vi "Demo.vi"() -> (4 "图像时间戳":u32=16532020 format="%_32g")   [LabVIEW 2012]
uses:
  MVCAMSDK.dll
panel:
  in  "自定义分辨率设置":bool
  in  "ROI分辨率":T1
  in  "预设分辨率设置":bool
  in  "预设分辨率":T2(radio)
  out "帧速":u32
  out "帧间耗时\n单位：（0.1ms）":u32
  in  "相机枚举":T3(ring)
  in  "自动曝光模式":bool=TRUE caption="软触发"
  in  "手动曝光模式":bool caption="软触发"
  in  "曝光时间，单位微秒":dbl=11000.0 format="%#_6f"
  in  "硬触发模式":bool caption="软触发"
  in  "软触发模式":bool caption="软触发"
  in  "连续模式":bool caption="软触发"
  in  "软触发一帧":bool caption="软触发"
  in  "读取自定义数据":bool
  out "从相机中读出的字符串(32字节)":string
  in  "写入自定义数据":bool
  in  "要写入相机的字符串(32字节)":string
  in  "拍照":bool
  in  "相机参数":bool=TRUE
  in  "Stop":bool
  in  "激活预览":bool=TRUE
  out "Image":T4(plugin-control)
  # "写入自定义数据"
  # "相机原生分辨率设置"
  # "触发设置"
  # "曝光设置"
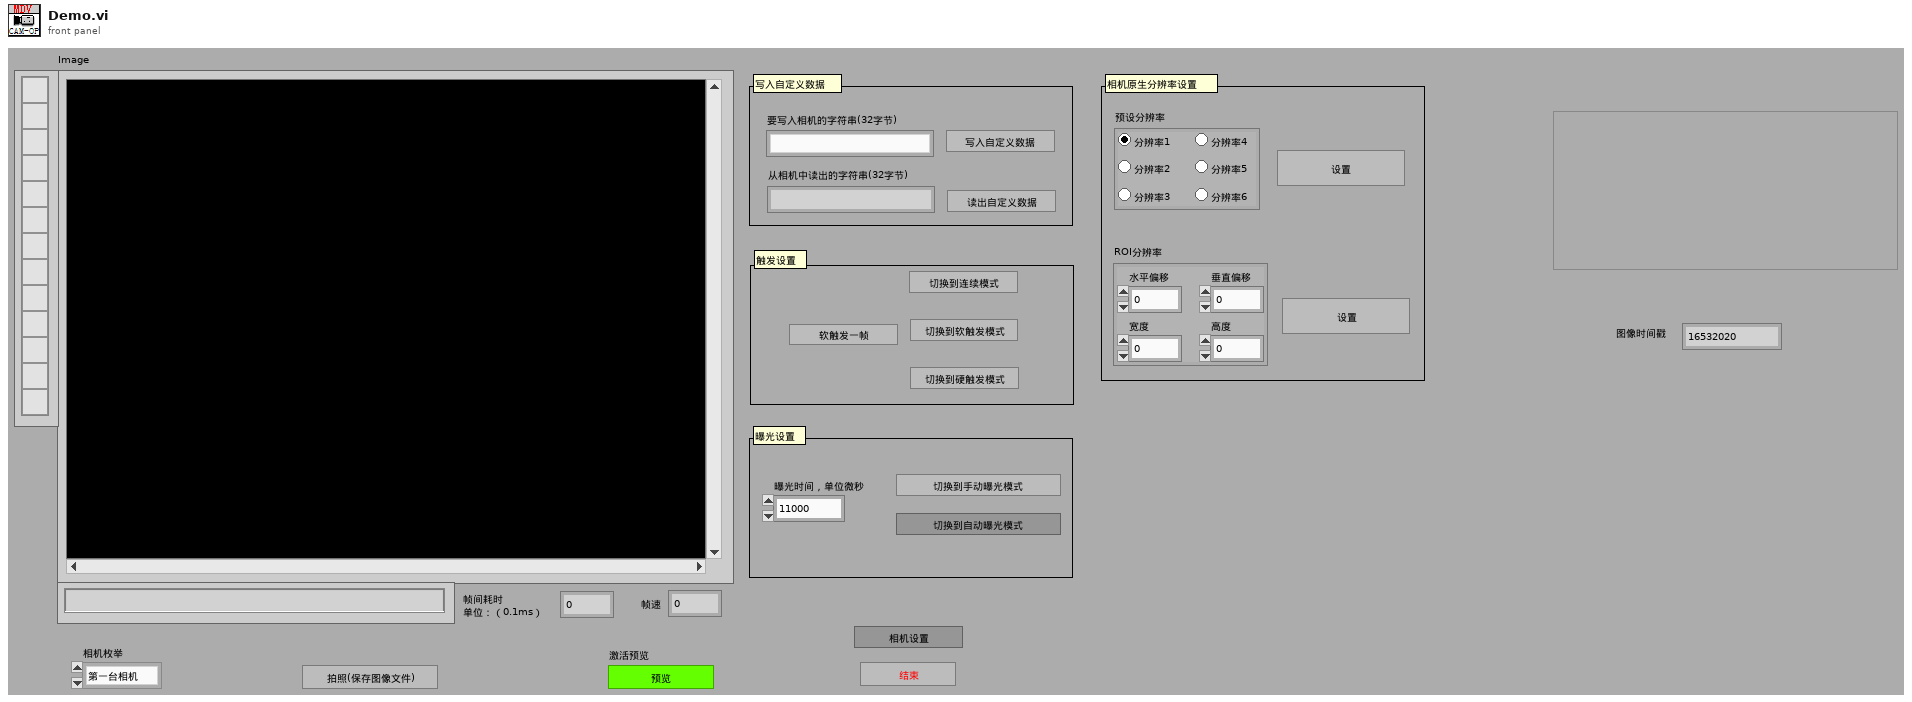
[diagram p1: front panel]
types:
  T1 = cluster{"水平偏移":dbl, "垂直偏移":dbl, "宽度":dbl, "高度":dbl}
  T2 = enum32{"分辨率1", "分辨率2", "分辨率3", "分辨率4", "分辨率5", "分辨率6"}
  T3 = enum16{"第一台相机", "第二台相机", "第三台相机", "第四台相机", "第五台相机"}
  T4 = typedef "IMAQ Image.ctl" = refnum<image>
  T5 = typedef "Image Type" = u32
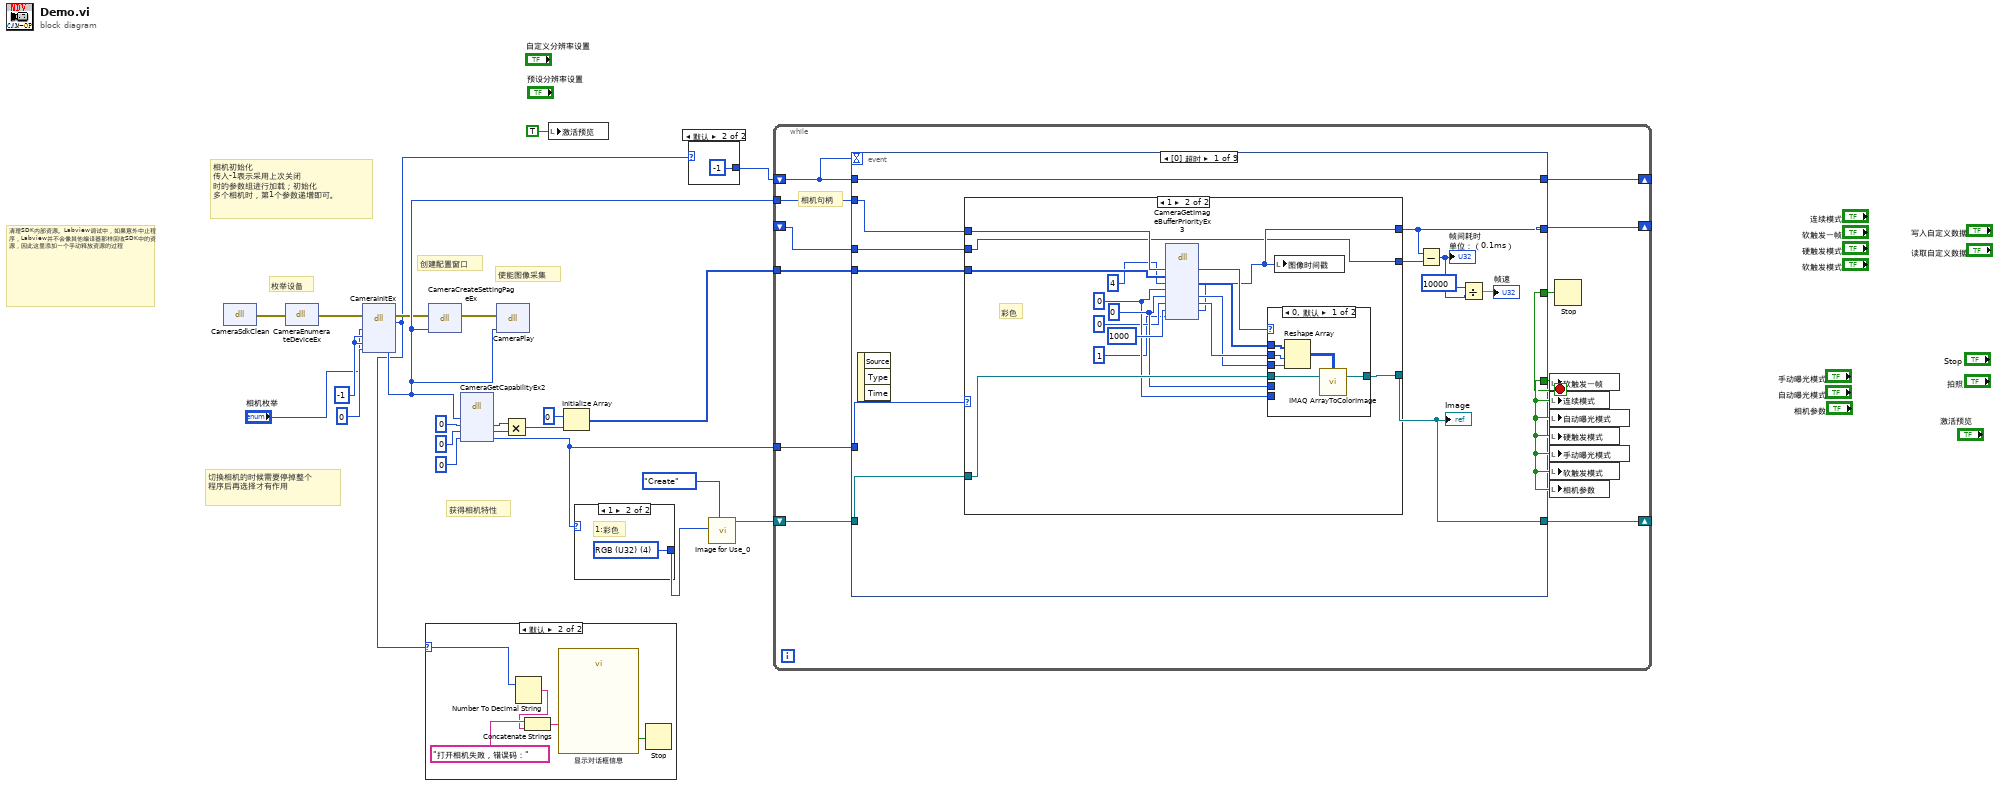
[diagram p0: block diagram]
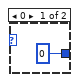
[diagram p2: hidden frame]
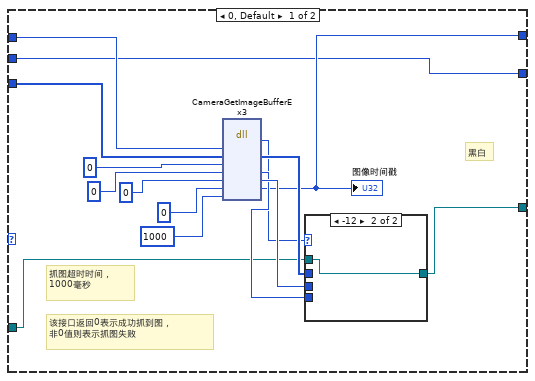
[diagram p4: hidden frame]
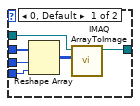
[diagram p5: hidden frame]
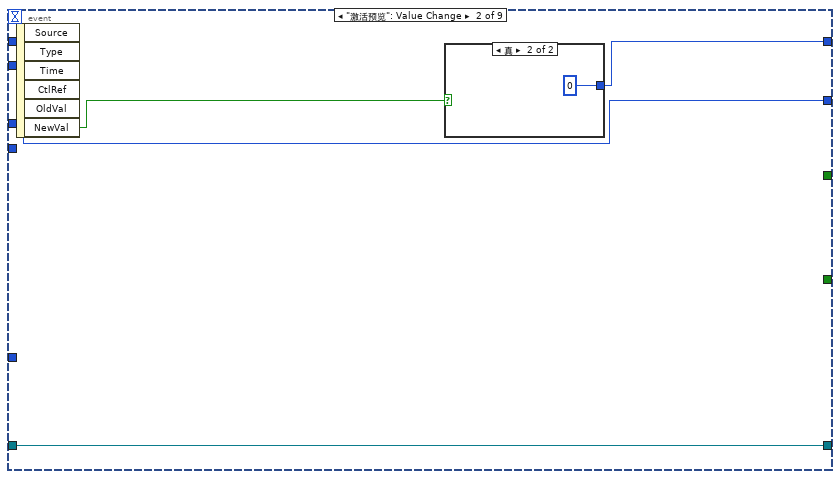
[diagram p7: hidden frame]
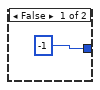
[diagram p8: hidden frame]
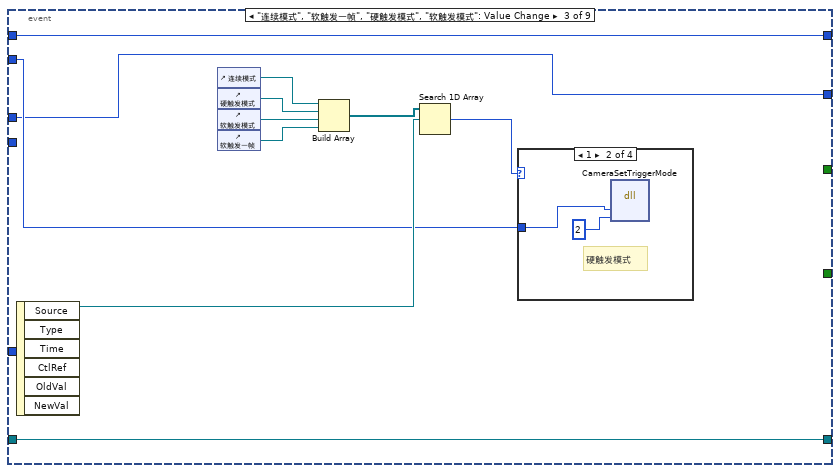
[diagram p9: hidden frame]
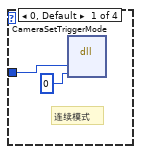
[diagram p10: hidden frame]
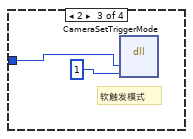
[diagram p11: hidden frame]
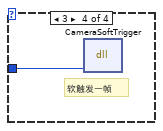
[diagram p12: hidden frame]
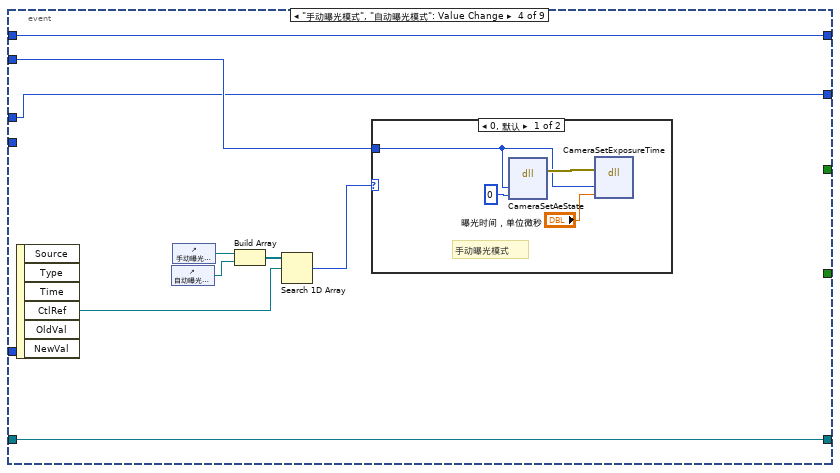
[diagram p13: hidden frame]
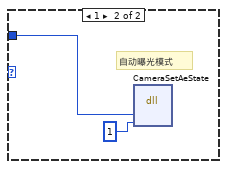
[diagram p14: hidden frame]
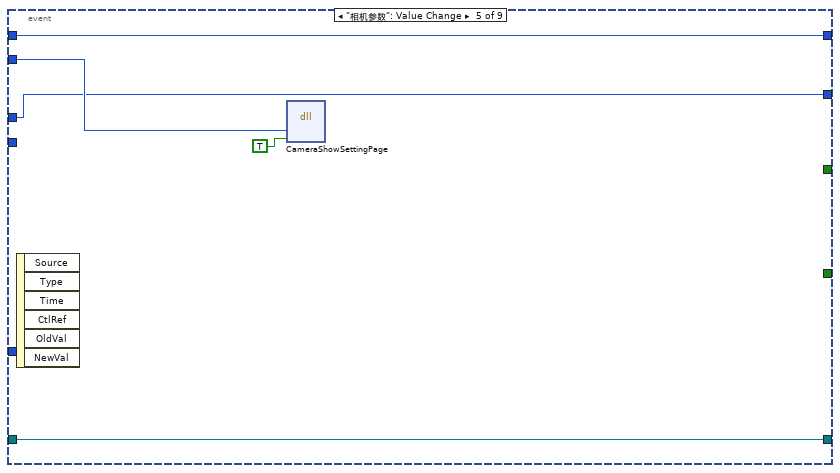
[diagram p15: hidden frame]
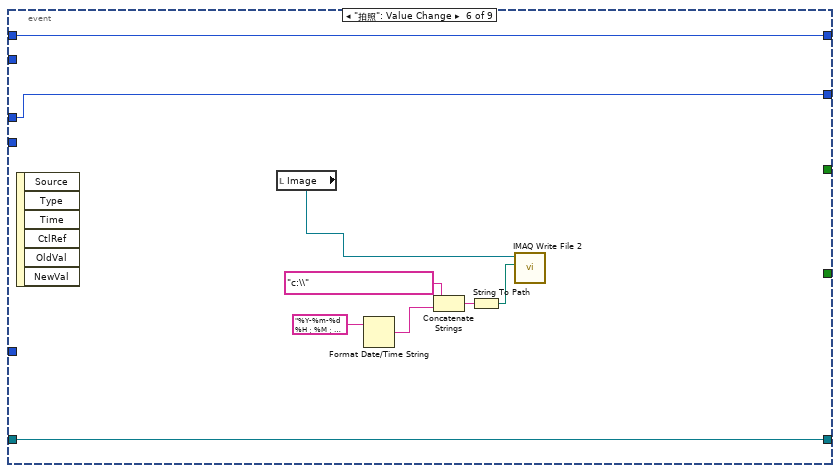
[diagram p16: hidden frame]
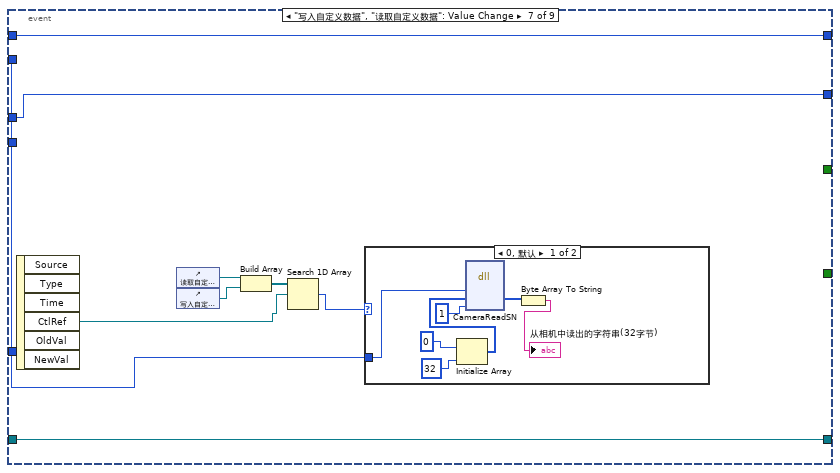
[diagram p17: hidden frame]
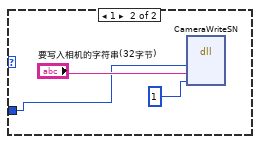
[diagram p18: hidden frame]
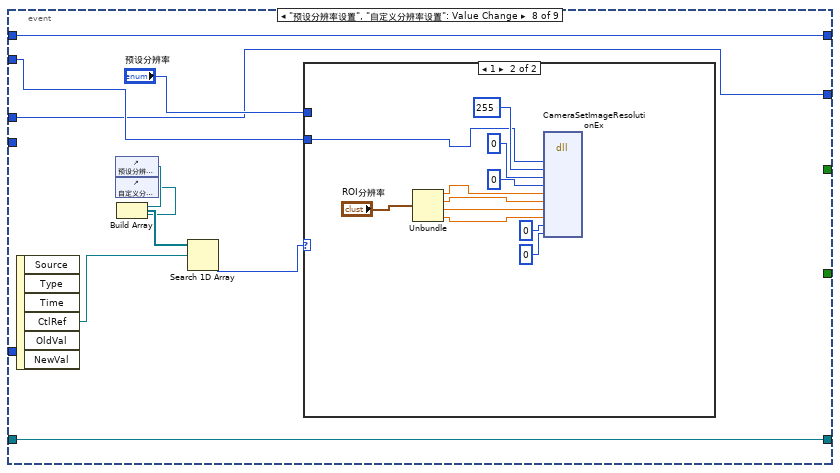
[diagram p19: hidden frame]
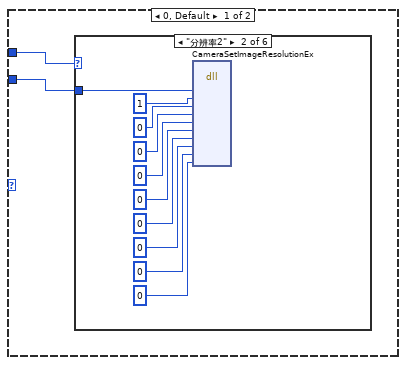
[diagram p20: hidden frame]
diagram:
  w20 = -1
  # "切换相机的时候需要停掉整个\n程序后再选择才有作用"
  # "清理SDK内部资源。Labview调试中，如果意外中止程序，Labview并不会像其他编译器那样回收SDK中的资源，因此这里添加一个手动释放资源的过程"
  # "使能图像采集"
  # "获得相机特性"
  # "创建配置窗口"
  # "相机初始化\n传入-1表示采用上次关闭\n时的参数组进行加载；初始化\n多个相机时，第1个参数递增即可。"
  # "枚举设备"
  n1 = dll-call lib="MVCAMSDK.dll" fn="CameraSdkClean"() -> (error out=w21:errorcluster)  [unwired: 4 in, 1 out]
  n2 = dll-call lib="MVCAMSDK.dll" fn="CameraEnumerateDeviceEx"(error in=w21) -> (error out=w18:errorcluster)  [unwired: 3 in, 1 out]
  n3 = dll-call lib="MVCAMSDK.dll" fn="CameraInitEx"(error in=w18, "相机索引值"="相机枚举", "参数加载方式"=w20, "要加载的参数组索引"=w20, "相机句柄"=0) -> (error out=w7:errorcluster, "返回类型"=w2:i32, "相机句柄"=w9:i32)  [unwired: 5 in, 1 out]
  n4 = case shown="默认" w2 {
    selector: w2 -> [_ w27]
    frame 0 {
    }
    frame Default {
      n5 = Number To Decimal String(number=w27) -> (decimal integer string=w24:string)  [unwired: 1 in]
      n6 = Concatenate Strings("打开相机失败，错误码：" ("字符串"), w24) -> (w26:string)
      n7 = call "显示对话框信息"("Message"=w26) -> ("结束"=w28:bool)  [unwired: 9 in, 1 out]
      n8 = Stop(stop? (T)=w28) -> ()
    }
  }
  n9 = dll-call lib="MVCAMSDK.dll" fn="CameraCreateSettingPageEx"(error in=w7, "相机句柄"=w9) -> (error out=w10:errorcluster)  [unwired: 4 in, 1 out]
  n10 = dll-call lib="MVCAMSDK.dll" fn="CameraGetCapabilityEx2"("相机句柄"=w9, "图像最大宽度"=0, "图像最大高度"=0, "是否是彩色相机(返回0:黑白;1:彩色)"=0) -> ("图像最大宽度"=w12:i32, "图像最大高度"=w11:i32, "是否是彩色相机(返回0:黑白;1:彩色)"=w6:i32)  [unwired: 5 in, 2 out]
  n11 = dll-call lib="MVCAMSDK.dll" fn="CameraPlay"(error in=w10, "相机句柄"=w9) -> ()  [unwired: 4 in, 2 out]
  n12 = Multiply(x=w12, y=w11) -> (x*y=w16:i32)
  n13 = local write "激活预览"(TRUE ("激活预览")) -> ()
  n14 = Initialize Array(0, w16) -> (w8:i32[])
  n15 = case shown="1" w6 {
    tunnel: [_ w29] -> w22
    frame 0, Default {
      # "0:黑白;"
    }
    frame 1 {
      w29 = T5 4 items=["Grayscale (U8)", "Grayscale (I16)", "Grayscale (SGL)", "Complex (CSG)", "RGB (U32)", "HSL (U32)", "RGB (U64)", "Grayscale (U16)"] ("Image Type")
      # "1:彩色"
    }
  }
  n16 = case shown="默认" w2 {
    tunnel: [0 -1] -> w1
    frame 0 {
    }
    frame Default {
    }
  }
  n17 = call "Image for Use_0.vi"("Command"=enum16{"Create", "Use", "Copy in", "Dispose"}."Create", "Image Type"=w22) -> ("Image out"=w5:T4)  [unwired: 8 in, 1 out]
  n18 = while {
    tunnel: w9 -> [w39]
    tunnel: w8 -> [w41]
    tunnel: w6 -> [w42]
    shift-right: [w38] -> _
    shift-left: w1 -> [w37]
    shift-right: [w35] -> _
    shift-left: w5 -> [w40]
    shift-right: [w34] -> _
    shift-left: _ -> [w33]
    stop <- w32 stop-if-true
    # "相机句柄"
    n19 = event shown="[0] 超时" {
      selector: _ -> [_ _ _ _ _ _ _ _ _]
      dyn-events: _ -> [_ _ _ _ _ _ _ _ _]
      timeout: w37 -> [_ _ _ _ _ _ _ _ _]
      tunnel: [_ _ _ _ _ _ _ _ TRUE] -> w32
      tunnel: w41 -> [w53 _ _ _ _ _ _ _ _]
      tunnel: w42 -> [w52 _ _ _ _ _ _ _ _]
      tunnel: w39 -> [w54 _ w108 w126 w141 _ w155 w178 w258]
      tunnel: w40 -> [w51 w101 w107 w125 w140 w145 w154 w180 w256]
      tunnel: [w50 w102 w109 w127 w142 w146 w156 w181 w259] -> w38
      tunnel: w37 -> [w50 _ w109 w127 w142 w146 w156 w181 w259]
      tunnel: [_ _ _ _ _ _ _ _ FALSE] -> w36
      tunnel: [w49 w101 w107 w125 w140 w145 w154 w180 w256] -> w35
      tunnel: [w46 w100 w106 w124 w139 w144 w153 w172 w255] -> w34
      tunnel: w33 -> [w48 w100 w106 w124 w139 w144 w153 w172 w255]
      event Timeout {
        n20 = event-data() -> ()  [unwired: 1 in, 3 out]
        n21 = case shown="1" w52 {
          tunnel: w53 -> [w69 w92]
          tunnel: w51 -> [w58 w91]
          tunnel: w54 -> [w57 w90]
          tunnel: [w59 w80] -> w49
          tunnel: [w56 w79] -> w46
          tunnel: w48 -> [w55 w78]
          tunnel: [w55 w78] -> w47
          frame 0, Default {
            # "黑白"
            # "该接口返回0表示成功抓到图，\n非0值则表示抓图失败"
            # "抓图超时时间，\n1000毫秒"
            n22 = dll-call lib="MVCAMSDK.dll" fn="CameraGetImageBufferEx3"("相机句柄"=w57, "图像数据缓冲区"=w69, "图像输出格式(0:8位灰度;1:24位彩色;2:32位彩色，3：BGR24彩色 4：BGRA32位彩色)"=0, "图像宽度"=0, "图像高度"=0, "时间戳(单位为100微秒)"=0, "抓图超时时间(毫秒)"=1000) -> ("返回类型"=w61:i32, "图像数据缓冲区"=w64:u8[], "图像宽度"=w62:i32, "图像高度"=w63:i32, "时间戳(单位为100微秒)"=w56:u32)  [unwired: 6 in, 2 out]
            "图像时间戳" <- w56
            n23 = case shown="-12" w61 {
              tunnel: w64 -> [w75 _]
              tunnel: w58 -> [w72 w76]
              tunnel: w63 -> [w74 _]
              tunnel: w62 -> [w73 _]
              tunnel: [w70 w76] -> w59
              frame 0, Default {
                n24 = Reshape Array(w75, w74, w73) -> (w71:u8[][])
                n25 = call "IMAQ ArrayToImage"("Image Pixels (U8)"=w71, "Image"=w72) -> ("Image Out"=w70:T4)  [unwired: 8 in, 1 out]
              }
              frame -12 {
              }
            }
          }
          frame 1 {
            w82 = 0
            w83 = 0
            # "彩色"
            n26 = dll-call lib="MVCAMSDK.dll" fn="CameraGetImageBufferPriorityEx3"("相机句柄"=w90, "图像数据缓冲区"=w92, "图像输出格式(0:8位灰度;1:24位彩色;2:32位彩色)"=4, "图像宽度"=w82, "图像高度"=w83, "时间戳（单位为100微秒）"=0, "抓图超时时间(毫秒)"=1000, "取图优先级(0: 取最旧   1:取最新)"=1) -> ("返回类型"=w84:i32, "图像数据缓冲区"=w87:u32[], "图像宽度"=w85:i32, "图像高度"=w86:i32, "时间戳（单位为100微秒）"=w79:u32)  [unwired: 7 in, 2 out]
            n27 = case shown="0, 默认" w84 {
              tunnel: w87 -> [w97 _]
              tunnel: w91 -> [w96 w99]
              tunnel: w86 -> [w95 _]
              tunnel: w85 -> [w94 _]
              tunnel: w83 -> [_ _]
              tunnel: w82 -> [_ _]
              tunnel: [w93 w99] -> w80
              frame 0, Default {
                n28 = Reshape Array(w97, w95, w94) -> (w98:u32[][])
                n29 = call "IMAQ ArrayToColorImage"("Image Pixels (U32)"=w98, "Image"=w96) -> ("Image Out"=w93:T4)  [unwired: 3 in, 1 out]
              }
              frame -12 {
              }
            }
            n30 = local write "图像时间戳"(w79) -> ()
          }
        }
        "Image" <- w49
        n31 = Subtract(x=w46, y=w47) -> (x-y=w45:u32)
        "帧间耗时\n单位：（0.1ms）" <- w45
        n32 = Divide(x=u32 10000 ("帧间耗时"), y=w45) -> (x/y=→"帧速":dbl)
      }
      event "激活预览": Value Change {
        n33 = event-data() -> ("NewVal"=w103:bool)  [unwired: 1 in, 5 out]
        n34 = case shown="真" w103 {
          tunnel: [-1 0] -> w102
          frame False {
          }
          frame True {
          }
        }
      }
      event "连续模式", "软触发一帧", "硬触发模式", "软触发模式": Value Change {
        n35 = event-data() -> ("CtlRef"=w111:refnum<vi>)  [unwired: 1 in, 5 out]
        n36 = control-ref of="连续模式"() -> (w113:refnum<vi>)
        n37 = control-ref of="硬触发模式"() -> (w114:refnum<vi>)
        n38 = control-ref of="软触发模式"() -> (w115:refnum<vi>)
        n39 = control-ref of="软触发一帧"() -> (w116:refnum<vi>)
        n40 = Build Array ("创建数组")(w113, w114, w115, w116) -> (w112:refnum<vi>[])
        n41 = Search 1D Array(1D array=w112, element=w111) -> (index of element=w110:i32)  [unwired: 1 in]
        n42 = case shown="1" w110 {
          tunnel: w108 -> [w117 w119 w121 w123]
          frame 0, Default {
            # "连续模式"
            n43 = dll-call lib="MVCAMSDK.dll" fn="CameraSetTriggerMode"("相机句柄"=w117, "模式"=0) -> ()  [unwired: 6 in, 2 out]
          }
          frame 1 {
            # "硬触发模式"
            n44 = dll-call lib="MVCAMSDK.dll" fn="CameraSetTriggerMode"("相机句柄"=w119, "模式"=2) -> ()  [unwired: 6 in, 2 out]
          }
          frame 2 {
            # "软触发模式"
            n45 = dll-call lib="MVCAMSDK.dll" fn="CameraSetTriggerMode"("相机句柄"=w121, "模式"=1) -> ()  [unwired: 6 in, 2 out]
          }
          frame 3 {
            # "软触发一帧"
            n46 = dll-call lib="MVCAMSDK.dll" fn="CameraSoftTrigger"("相机句柄"=w123) -> ()  [unwired: 5 in, 2 out]
          }
        }
      }
      event "手动曝光模式", "自动曝光模式": Value Change {
        n47 = event-data() -> ("CtlRef"=w130:refnum<vi>)  [unwired: 1 in, 5 out]
        n48 = control-ref of="自动曝光模式"() -> (w128:refnum<vi>)
        n49 = control-ref of="手动曝光模式"() -> (w131:refnum<vi>)
        n50 = Build Array ("创建数组")(w131, w128) -> (w132:refnum<vi>[])
        n51 = Search 1D Array(1D array=w132, element=w130) -> (index of element=w129:i32)  [unwired: 1 in]
        n52 = case shown="0, 默认" w129 {
          tunnel: w126 -> [w133 w137]
          frame 0, Default {
            # "手动曝光模式"
            n53 = dll-call lib="MVCAMSDK.dll" fn="CameraSetAeState"("相机句柄"=w133, "曝光模式(0手动，1自动)"=0) -> (error out=w136:errorcluster)  [unwired: 6 in, 1 out]
            n54 = dll-call lib="MVCAMSDK.dll" fn="CameraSetExposureTime"(error in=w136, "相机句柄"=w133, "曝光时间，单位微秒"="曝光时间，单位微秒") -> ()  [unwired: 5 in, 2 out]
          }
          frame 1 {
            # "自动曝光模式"
            n55 = dll-call lib="MVCAMSDK.dll" fn="CameraSetAeState"("相机句柄"=w137, "曝光模式(0手动，1自动)"=1) -> ()  [unwired: 6 in, 2 out]
          }
        }
      }
      event "相机参数": Value Change {
        n56 = event-data() -> ()  [unwired: 1 in, 6 out]
        n57 = dll-call lib="MVCAMSDK.dll" fn="CameraShowSettingPage"("相机句柄"=w141, "状态"=TRUE) -> ()  [unwired: 6 in, 2 out]
      }
      event "拍照": Value Change {
        n58 = event-data() -> ()  [unwired: 1 in, 6 out]
        n59 = local read "Image"() -> (w147:T4)
        n60 = Format Date/Time String(time format string (%c)="%Y-%m-%d %H：%M：%S.bmp ") -> (date/time string=w151:string)  [unwired: 2 in]
        n61 = Concatenate Strings("c:\\", w151) -> (w148:string)
        n62 = String To Path(string=w148) -> (path=w150:path)
        n63 = call-poly "IMAQ Write File 2"("File Path"=w150, "Image"=w147) -> ()  [unwired: 8 in, 2 out]
      }
      event "写入自定义数据", "读取自定义数据": Value Change {
        n64 = event-data() -> ("CtlRef"=w158:refnum<vi>)  [unwired: 1 in, 5 out]
        n65 = control-ref of="读取自定义数据"() -> (w160:refnum<vi>)
        n66 = control-ref of="写入自定义数据"() -> (w159:refnum<vi>)
        n67 = Build Array ("创建数组")(w160, w159) -> (w161:refnum<vi>[])
        n68 = Search 1D Array(1D array=w161, element=w158) -> (index of element=w157:i32)  [unwired: 1 in]
        n69 = case shown="0, 默认" w157 {
          tunnel: w155 -> [w162 w169]
          frame 0, Default {
            n70 = Initialize Array(0, 32) -> (w166:i32[])
            n71 = dll-call lib="MVCAMSDK.dll" fn="CameraReadSN"("相机句柄"=w162, "序列号"=w166, "序列号级别，[0,1,2],0级为只读，1,2级可写"=1) -> ("序列号"=w164:u8[])  [unwired: 6 in, 2 out]
            n72 = Byte Array To String(unsigned byte array=w164) -> (string=→"从相机中读出的字符串(32字节)":string)
          }
          frame 1 {
            n73 = dll-call lib="MVCAMSDK.dll" fn="CameraWriteSN"("相机句柄"=w169, "序列号(固定为32个字节)"="要写入相机的字符串(32字节)", "序列号级别，[0,1,2]对应3级序列号，其中0级为只读，1,2级可写"=1) -> ()  [unwired: 7 in, 2 out]
          }
        }
      }
      event "预设分辨率设置", "自定义分辨率设置": Value Change {
        n74 = event-data() -> ("CtlRef"=w174:refnum<vi>)  [unwired: 1 in, 5 out]
        n75 = control-ref of="预设分辨率设置"() -> (w176:refnum<vi>)
        n76 = control-ref of="自定义分辨率设置"() -> (w175:refnum<vi>)
        n77 = Build Array ("创建数组")(w176, w175) -> (w177:refnum<vi>[])
        n78 = Search 1D Array(1D array=w177, element=w174) -> (index of element=w173:i32)  [unwired: 1 in]
        n79 = case shown="1" w173 {
          tunnel: "预设分辨率" -> [w183 _]
          tunnel: w178 -> [w182 w244]
          frame 0, Default {
            n80 = case shown="\"分辨率2\"" w183 {
              tunnel: w182 -> [w184 w203 w204 w214 w224 w234]
              frame "分辨率1", Default {
                n81 = dll-call lib="MVCAMSDK.dll" fn="CameraSetImageResolutionEx"("相机句柄"=w184, "预设分辨率索引"=0, "Mode"=0, "ModeSize"=u32 0, "x"=0, "y"=u32 0 ("ModeSize"), "width"=0, "height"=0, "ZoomWidth"=0, "ZoomHeight"=0) -> ()  [unwired: 14 in, 2 out]
              }
              frame "分辨率2" {
                n82 = dll-call lib="MVCAMSDK.dll" fn="CameraSetImageResolutionEx"("相机句柄"=w203, "预设分辨率索引"=1, "Mode"=0, "ModeSize"=u32 0, "x"=0, "y"=u32 0 ("ModeSize"), "width"=0, "height"=0, "ZoomWidth"=0, "ZoomHeight"=0) -> ()  [unwired: 14 in, 2 out]
              }
              frame "分辨率3" {
                n83 = dll-call lib="MVCAMSDK.dll" fn="CameraSetImageResolutionEx"("相机句柄"=w204, "预设分辨率索引"=2, "Mode"=0, "ModeSize"=u32 0, "x"=0, "y"=u32 0 ("ModeSize"), "width"=0, "height"=0, "ZoomWidth"=0, "ZoomHeight"=0) -> ()  [unwired: 14 in, 2 out]
              }
              frame "分辨率4" {
                n84 = dll-call lib="MVCAMSDK.dll" fn="CameraSetImageResolutionEx"("相机句柄"=w214, "预设分辨率索引"=3, "Mode"=0, "ModeSize"=u32 0, "x"=0, "y"=u32 0 ("ModeSize"), "width"=0, "height"=0, "ZoomWidth"=0, "ZoomHeight"=0) -> ()  [unwired: 14 in, 2 out]
              }
              frame "分辨率5" {
                n85 = dll-call lib="MVCAMSDK.dll" fn="CameraSetImageResolutionEx"("相机句柄"=w224, "预设分辨率索引"=4, "Mode"=0, "ModeSize"=u32 0, "x"=0, "y"=u32 0 ("ModeSize"), "width"=0, "height"=0, "ZoomWidth"=0, "ZoomHeight"=0) -> ()  [unwired: 14 in, 2 out]
              }
              frame "分辨率6" {
                n86 = dll-call lib="MVCAMSDK.dll" fn="CameraSetImageResolutionEx"("相机句柄"=w234, "预设分辨率索引"=5, "Mode"=0, "ModeSize"=u32 0, "x"=0, "y"=u32 0 ("ModeSize"), "width"=0, "height"=0, "ZoomWidth"=0, "ZoomHeight"=0) -> ()  [unwired: 14 in, 2 out]
              }
            }
          }
          frame 1 {
            n87 = Unbundle("ROI分辨率") -> ("水平偏移"=w246:dbl, "垂直偏移"=w247:dbl, "宽度"=w248:dbl, "高度"=w249:dbl)
            n88 = dll-call lib="MVCAMSDK.dll" fn="CameraSetImageResolutionEx"("相机句柄"=w244, "预设分辨率索引"=255, "Mode"=0, "ModeSize"=u32 0, "x"=w246, "y"=w247, "width"=w248, "height"=w249, "ZoomWidth"=0, "ZoomHeight"=u32 0 ("ModeSize")) -> ()  [unwired: 14 in, 2 out]
          }
        }
      }
      event "Stop": Value Change {
        # "反初始化相机"
        n89 = event-data() -> ()  [unwired: 1 in, 6 out]
        n90 = dll-call lib="MVCAMSDK.dll" fn="CameraUnInit"("相机句柄"=w258) -> ()  [unwired: 5 in, 2 out]
      }
    }
    n91 = local write "软触发一帧"(w36) -> ()
    n92 = local write "连续模式"(w36) -> ()
    n93 = local write "自动曝光模式"(w36) -> ()
    n94 = local write "硬触发模式"(w36) -> ()
    n95 = local write "手动曝光模式"(w36) -> ()
    n96 = local write "软触发模式"(w36) -> ()
    n97 = local write "相机参数"(w36) -> ()
    n98 = Stop(stop? (T)=w32) -> ()
  }
